vi "DrawTiles.vi"(8 "error in (no error)":errorcluster, 11 "Game in":refnum<class "Game.lvclass">) -> (0 "error out":errorcluster, 3 "Game out":refnum<class "Game.lvclass">)   [LabVIEW 2019, in "RT_Game.lvlib" / "Game.lvclass"]
uses:
  Game.lvclass
  Game.lvclass/Game.ctl
  <vilib>/Utility/error.llb/Error Cluster From Error Code.vi
  <vilib>/rvi/errors/niLvFpgaAdjustHostInterfaceError.vi
  <vilib>/rvi/interface/nirviMethod/nirviMethod.xnode
  FPGA_Interface.ctl
  FPGA Bitfiles/myriogameconsole_FPGATarget_Main_ntsPRcBZGxk.lvbitx
  <vilib>/FPGAPlugInAG/myRIO-1900/niLvFpga_WriteFifo_myRIO-1900.vi
  <vilib>/rvi/errors/niLvFpgaMergeErrorWithErrorCode.vi
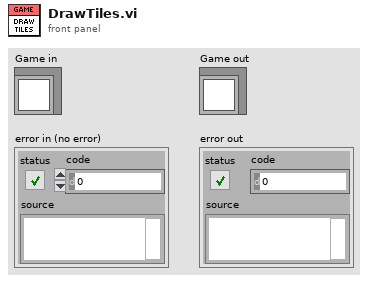
[diagram p1: front panel]
types:
  T1 = typedef "FPGA_Interface.ctl" = refnum<k20>
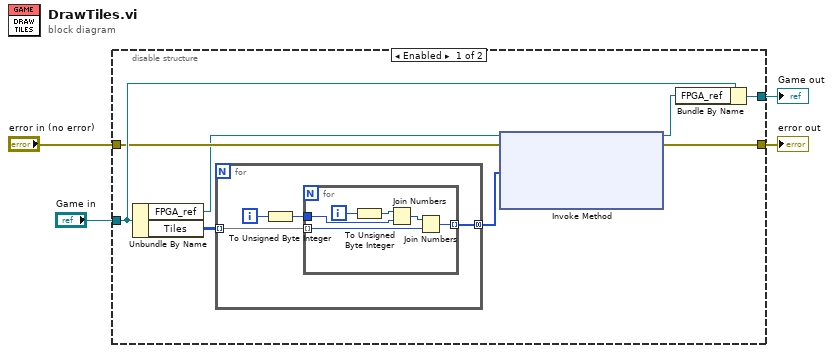
[diagram p0: block diagram]
diagram:
  n1 = disable-structure shown="Enabled" {
    disable-tunnel: [w12 w24] -> w4
    disable-tunnel: "Game in" -> [w11 w24]
    disable-tunnel: [w10 w23] -> w2
    disable-tunnel: "error in (no error)" -> [w9 w23]
    frame Enabled {
      n2 = Unbundle By Name(w11) -> ("FPGA_ref"=w5:T1, "Tiles"=w6:u16[][])
      n3 = for {
        tunnel: w6 -> [w16] mode=indexing
        tunnel: [w15] -> w7 mode=concatenating
        i -> [w14]
        n4 = To Unsigned Byte Integer(number=w14) -> (unsigned 8bit integer=w13:u8)
        n5 = for {
          tunnel: w16 -> [w17] mode=indexing
          tunnel: [w22] -> w15 mode=indexing
          tunnel: w13 -> [w20]
          i -> [w21]
          n6 = To Unsigned Byte Integer(number=w21) -> (unsigned 8bit integer=w18:u8)
          n7 = Join Numbers(hi=w18, lo=w20) -> ((hi.lo)=w19:u16)
          n8 = Join Numbers(hi=w19, lo=w17) -> ((hi.lo)=w22:u32)
        }
      }
      n9 = xnode "Invoke Method"("FPGA VI Reference In"=w5, "error in"=w9, "Data"=w7) -> ("FPGA VI Reference Out"=w8:T1, "error out"=w10:errorcluster)  [unwired: 1 in, 1 out]
      n10 = Bundle By Name(cluster=w11, "FPGA_ref"=w8) -> (w12:refnum<class "Game.lvclass">)
    }
    frame Disabled {
    }
  }
  "Game out" <- w4
  "error out" <- w2
